vi "General Gauss-Mod Sine.vi"(4 "attenuation":dbl=6.0, 5 "X":dbl[](array[numeric]), 6 "bandwidth":dbl=0.15, 7 "center frequency":dbl=1.0, 8 "delta t":dbl=0.1, 9 "delay":dbl, 10 "amplitude":dbl=1.0, 11 "samples":i32=128) -> (0 "error":i32, 3 "Gauss-Mod Sine Pattern":dbl[](array[numeric]))   [LabVIEW 2017, in "NI_AALBase.lvlib"]
uses:
  <vilib>/Analysis/NI_AALBase.lvlib
  <resource>/lvanlys.dll
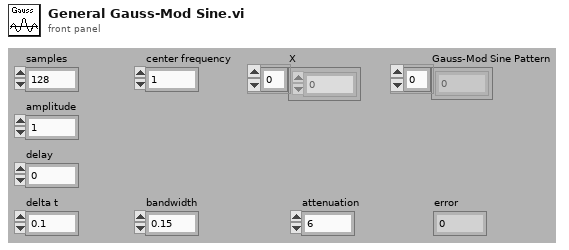
[diagram p1: front panel]
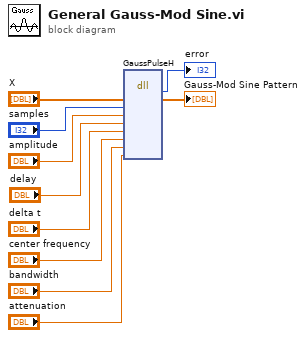
[diagram p0: block diagram]
diagram:
  n1 = dll-call lib="e:/builds/penguin/labview/branches/2017/dev/dist/resource/lvanlys.*" fn="GaussPulseH"("x"="X", "samples"="samples", "amplitude"="amplitude", "delay"="delay", "delta"="delta t", "fc"="center frequency", "bw"="bandwidth", "bwr"="attenuation") -> ("error"=→"error":i32, "x"=→"Gauss-Mod Sine Pattern":dbl[])  [unwired: 10 in, 2 out]
